vi "Process.vi"(8 "error in (no error)":errorcluster, 11 "USB DAQ in":refnum<class "USB DAQ.lvclass">) -> (0 "error out":errorcluster, 3 "USB DAQ out":refnum<class "USB DAQ.lvclass">)   [LabVIEW 2025, in "USB DAQ.lvclass"]
uses:
  USB DAQ.lvclass
  USB DAQ.lvclass/USB DAQ.ctl
  <vilib>/Handler Framework/Handler Framework.lvlib
  <vilib>/Handler Framework/CmdQueue/Enqueue Single.vi
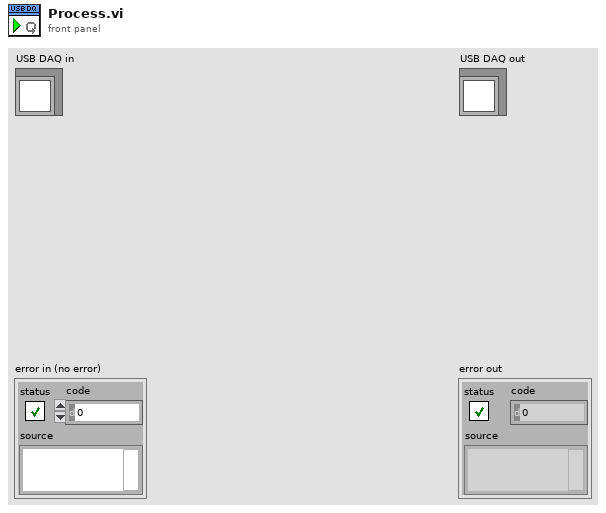
[diagram p1: front panel]
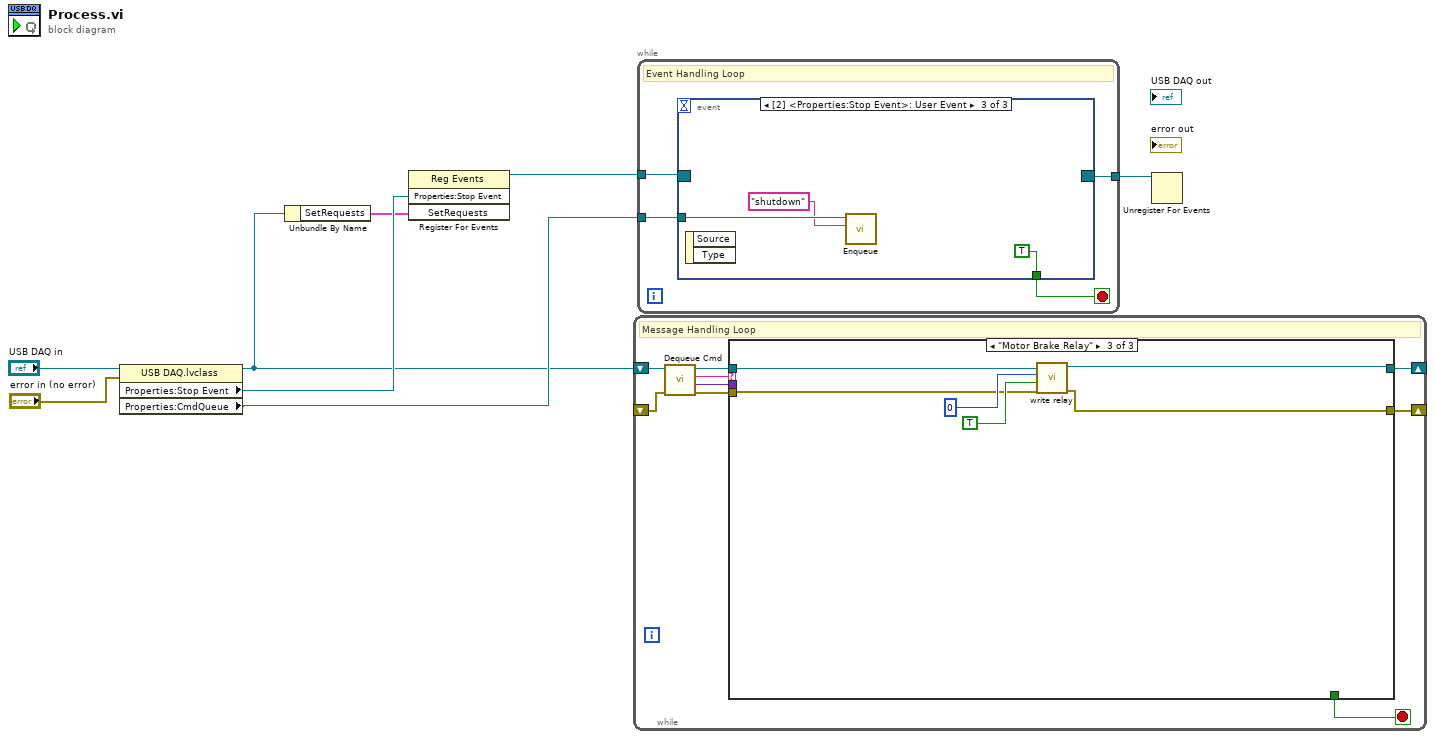
[diagram p0: block diagram]
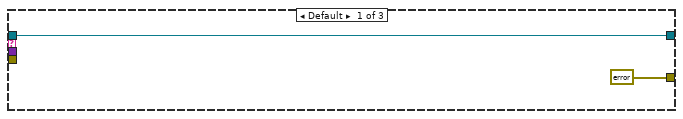
[diagram p2: hidden frame]
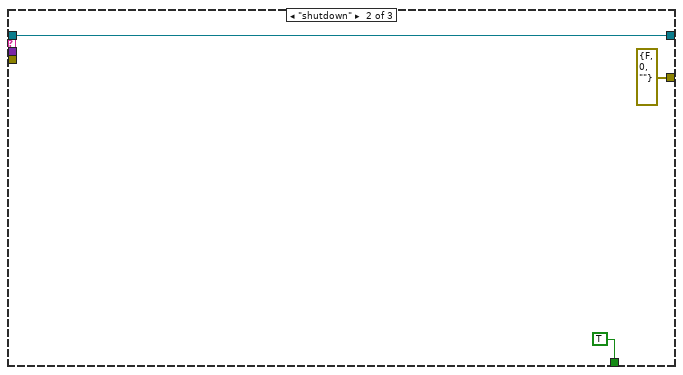
[diagram p3: hidden frame]
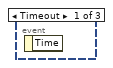
[diagram p4: hidden frame]
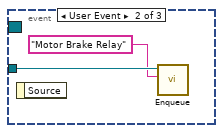
[diagram p5: hidden frame]
diagram:
  n1 = property class="USB DAQ.lvclass"(reference="USB DAQ in", error in="error in (no error)") -> (reference out=w1:refnum<class "USB DAQ.lvclass">, "Properties:Stop Event"=w6:refnum<user-event>, "Properties:CmdQueue"=w2:refnum<queue>)  [unwired: 1 out]
  n2 = Unbundle By Name(w1) -> ("SetRequests"=w4:cluster{"Motor Brake Relay":refnum<user-event>})
  n3 = register-events(w6, w4) -> (reference out=w5:refnum<event-registration>)  [unwired: 2 in, 1 out]
  n4 = while {
    shift-right: [w11] -> _
    shift-left: _ -> [w16]
    shift-right: [w12] -> _
    shift-left: w1 -> [w17]
    stop <- w10 stop-if-true
    # "Message Handling Loop"
    n5 = call-dynamic "Dequeue Cmd.vi"("error in (no error)"=w16, "Handler in"=w17) -> ("error out"=w9:errorcluster, "value"=w14:variant, "cmd"=w15:string, "Handler out"=w13:refnum<class "USB DAQ.lvclass">)  [unwired: 5 in, 1 out]
    n6 = case shown="\"Motor Brake Relay\"" w15 {
      tunnel: w14 -> [_ _ _]
      tunnel: w13 -> [w19 w21 w28]
      tunnel: [w19 w21 w25] -> w12
      tunnel: [errorcluster {"status"=FALSE, "code"=0, "source"=""} ("error in (no error)") errorcluster {"status"=FALSE, "code"=0, "source"=""} ("error in (no error)") w24] -> w11
      tunnel: [_ TRUE _] -> w10
      tunnel: w9 -> [_ _ w23]
      frame Default {
      }
      frame "shutdown" {
      }
      frame "Motor Brake Relay" {
        n7 = call-dynamic "write relay.vi"("error in (no error)"=w23, "value"=TRUE, "index"=0, "USB DAQ in"=w28) -> ("error out"=w24:errorcluster, "USB DAQ out"=w25:refnum<class "USB DAQ.lvclass">)  [unwired: 6 in]
      }
    }
  }
  n8 = while {
    tunnel: w5 -> [w32]
    tunnel: [w31] -> w3
    tunnel: w2 -> [w30]
    stop <- w29 stop-if-true
    # "Event Handling Loop"
    n9 = event shown="[2] <Properties:Stop Event>: User Event" {
      selector: w32 -> [_ _ _]
      dyn-events: [_ _ _] -> w31
      timeout: _ -> [_ _ _]
      tunnel: w30 -> [_ w34 w36]
      tunnel: [_ _ TRUE] -> w29
      event Timeout {
        n10 = event-data() -> ()  [unwired: 1 in, 1 out]
      }
      event User Event {
        n11 = event-data() -> ()  [unwired: 1 in, 1 out]
        n12 = call-poly <vilib>:"Enqueue.vi"("Command"="Motor Brake Relay", "CmdQueue in"=w34) -> ()  [unwired: 8 in, 2 out]
      }
      event User Event {
        n13 = event-data() -> ()  [unwired: 1 in, 2 out]
        n14 = call-poly <vilib>:"Enqueue.vi"("Command"="shutdown", "CmdQueue in"=w36) -> ()  [unwired: 8 in, 2 out]
      }
    }
  }
  n15 = Unregister For Events(event registration refnum=w3) -> ()  [unwired: 1 in, 1 out]
